vi "GEA2 Register Source Address.vi"(5 "Old Address":u8, 7 "New Address":u8, 11 "Error In":errorcluster) -> (15 "Error Out":errorcluster)   [LabVIEW 2016, in "GEA2_Toolkit.lvlib"]
doc: "This VI unregisters the address you specify and registers a new address on the GEA2 bus."
uses:
  library/GEA2_Toolkit.lvlib
  C:/Technology Lab/NI-2010/Trunk/Utility/LabVIEW GEA2 Toolkit v1.0.0.0/Appliance.NET/GeaCommunication.dll
  Appliance.NET/GeaCommunication.dll
panel:
  out "GEA2 Reference Out":refnum<k24>
  in  "GEA2 Reference In":refnum<k24>
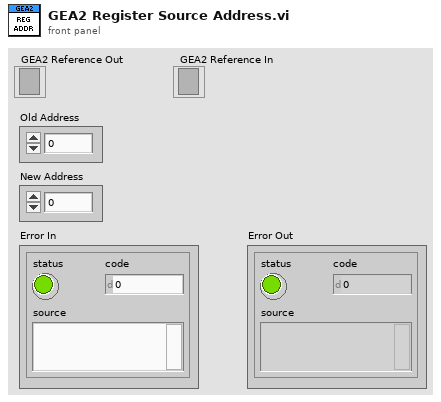
[diagram p1: front panel]
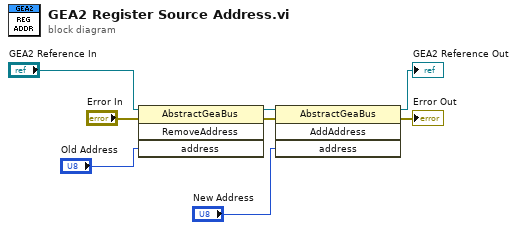
[diagram p0: block diagram]
diagram:
  n1 = invoke class="AbstractGeaBus" method="RemoveAddress"(reference="GEA2 Reference In", error in="Error In", "address"="Old Address") -> (reference out=w6:refnum<k24>, error out=w7:errorcluster)  [unwired: 1 in, 2 out]
  n2 = invoke class="AbstractGeaBus" method="AddAddress"(reference=w6, error in=w7, "address"="New Address") -> (reference out=→"GEA2 Reference Out":refnum<k24>, error out=→"Error Out":errorcluster)  [unwired: 1 in, 2 out]
